vi "Test Connection.vi"() -> ()   [LabVIEW 2020]
uses:
  <vilib>/LabVIEW Open Source Project/MQTT Client/Client class/Client.lvclass
  <vilib>/LabVIEW Open Source Project/MQTT Connection/MQTT_Base/Base Class/MQTT_Base.lvclass
  <vilib>/LabVIEW Open Source Project/MQTT Control Packets/Control Packets/PUBLISH/PUBLISH.lvclass
  <vilib>/LabVIEW Open Source Project/MQTT Control Packets/Control Packets/ControlPacket/ControlPacket.lvclass
  <vilib>/LabVIEW Open Source Project/Connection/Connection.TCP/Connection.TCP.lvclass
  <vilib>/LabVIEW Open Source Project/Connection/Connection.LocalQueue/Connection.LocalQueue.lvclass
  <vilib>/LabVIEW Open Source Project/Connection/Connection/Connection.lvclass
  <vilib>/LabVIEW Open Source Project/MQTT Control Packets/Control Packets/CONNECT/ConnectFlags -- cluster.ctl
  <vilib>/LabVIEW Open Source Project/MQTT Control Packets/Control Packets/CONNECT/CONNECT.lvclass
  Class/SecureMqttCodec/SecureMqttCodec.lvclass
  <vilib>/LabVIEW Open Source Project/MQTT Control Packets/Control Packets/ControlPacket/QualityOfService -- enum.ctl
  C:/Program Files/National Instruments/LabVIEW 2020/vi.lib/LabVIEW Open Source Project/Connection/Connection/Connection.lvclass
  C:/Program Files/National Instruments/LabVIEW 2020/vi.lib/LabVIEW Open Source Project/Connection/Connection.TCP/Connection.TCP.lvclass
  C:/Program Files/National Instruments/LabVIEW 2020/vi.lib/LabVIEW Open Source Project/MQTT Connection/MQTT_Base/Base Class/MQTT_Base.lvclass
  C:/Program Files/National Instruments/LabVIEW 2020/vi.lib/LabVIEW Open Source Project/MQTT Client/Client class/Client.lvclass
  C:/Program Files/National Instruments/LabVIEW 2020/vi.lib/LabVIEW Open Source Project/Connection/Connection.LocalQueue/Connection.LocalQueue.lvclass
  C:/Program Files/National Instruments/LabVIEW 2020/vi.lib/LabVIEW Open Source Project/MQTT Control Packets/Control Packets/ControlPacket/ControlPacket.lvclass
  C:/Program Files/National Instruments/LabVIEW 2020/vi.lib/LabVIEW Open Source Project/MQTT Control Packets/Control Packets/PUBLISH/PUBLISH.lvclass
panel:
  out "Incoming Message":u8[](array[numeric]) format="%08b"
  in  "Subscribe":bool
  out "Suback":bool
  out "Published":bool
  in  "Publish":bool
  in  "Stop Client":bool
  out "error out":errorcluster
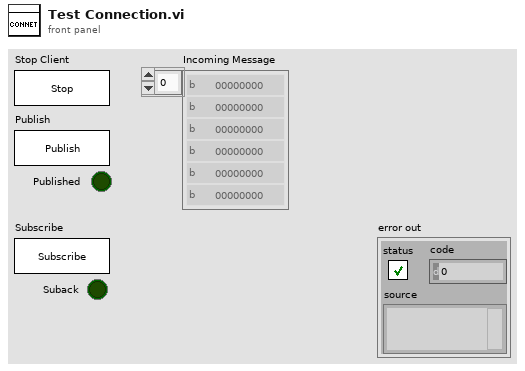
[diagram p1: front panel]
types:
  T1 = typedef "MQTT_Control_Packets.lvlib/CONNECT.lvclass/ConnectFlags -- cluster.ctl" = cluster{"Reserved":bool, "Clean Session":bool, "Will Flag":bool, "Will QoS 1":bool, "Will QoS 2":bool, "Will Retain":bool, "Password Flag":bool, "User Name Flag":bool}
  T2 = cluster{"Will Topic":string, "Will Message":string, "Username":string, "Password":string}
  T3 = typedef "MQTT Client.lvlib/Client.lvclass/Public Events -- cluster.ctl" = cluster{"Connection Status":refnum<user-event>, "Connected":refnum<user-event>, "Application Message":refnum<user-event>}
  T4 = typedef "MQTT Base.lvlib/MQTT_Base.lvclass/Public Events -- cluster.ctl" = cluster{"Stop Event":refnum<user-event>, "Error Event":refnum<user-event>, "Inbound Message":refnum<user-event>}
  T5 = typedef "MQTT_Control_Packets.lvlib/ControlPacket.lvclass/QualityOfService -- enum.ctl" = enum16{"0 (At Most Once)", "1 (At Least Once)", "2 (Exactly Once)"}
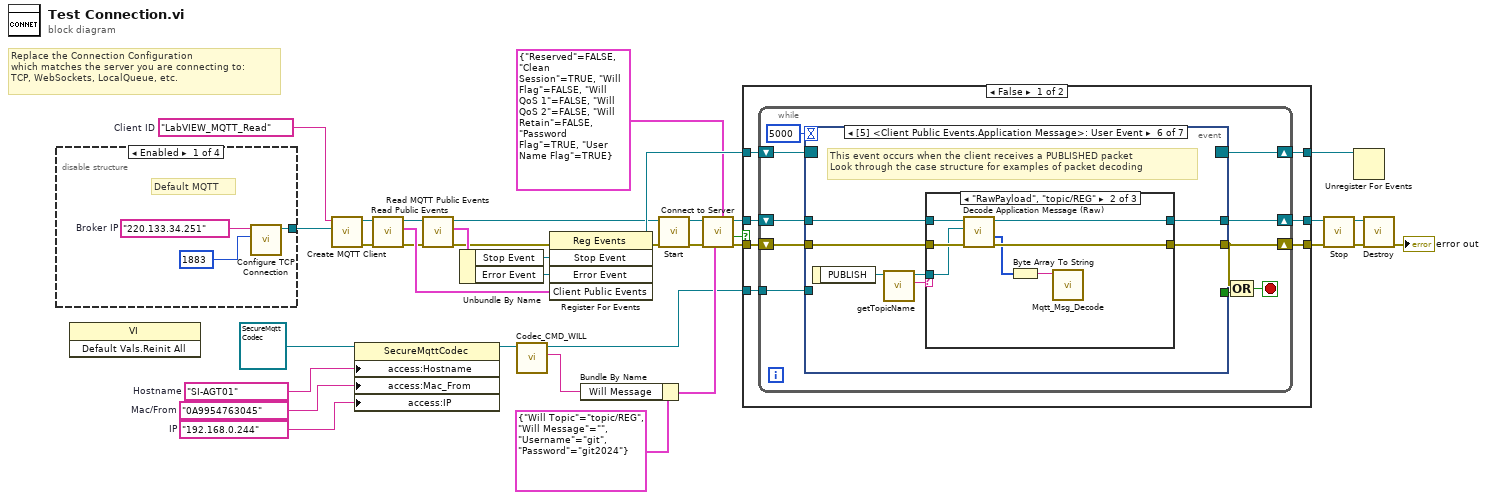
[diagram p0: block diagram]
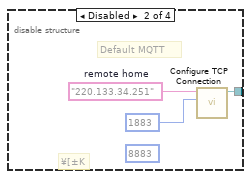
[diagram p2: hidden frame]
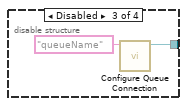
[diagram p3: hidden frame]
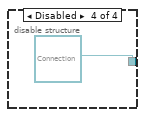
[diagram p4: hidden frame]
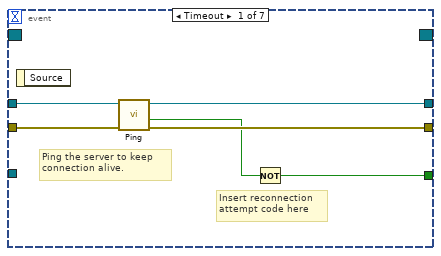
[diagram p5: hidden frame]
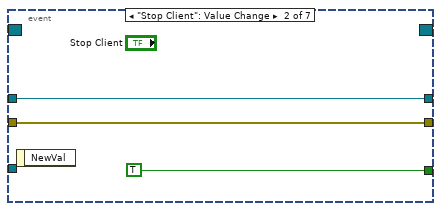
[diagram p6: hidden frame]
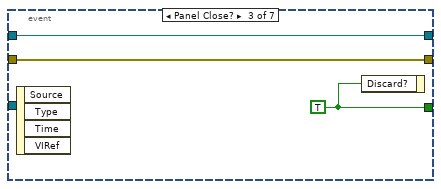
[diagram p7: hidden frame]
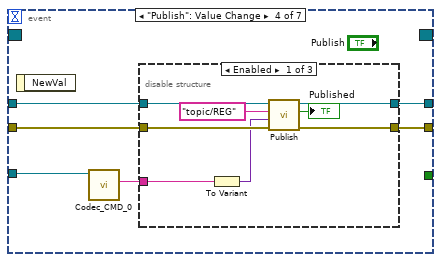
[diagram p8: hidden frame]
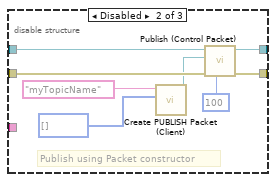
[diagram p9: hidden frame]
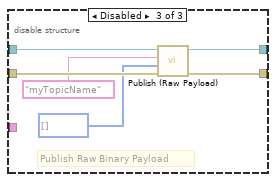
[diagram p10: hidden frame]
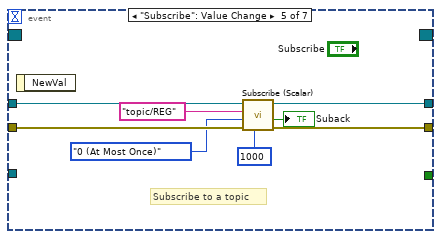
[diagram p11: hidden frame]
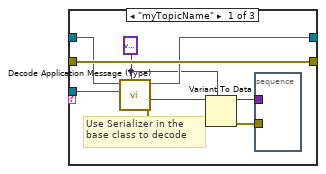
[diagram p12: hidden frame]
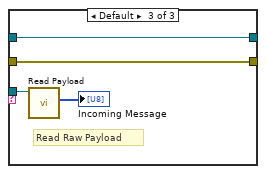
[diagram p13: hidden frame]
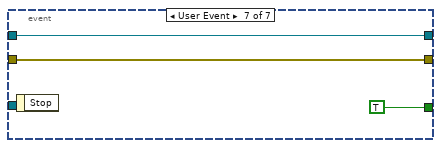
[diagram p14: hidden frame]
diagram:
  w1 = "192.168.0.244"  # IP
  w2 = "0A9954763045"  # Mac/From
  w3 = "SI-AGT01"  # Hostname
  w9 = "LabVIEW_MQTT_Read"  # Client ID
  # "Replace the Connection Configuration\nwhich matches the server you are connecting to:\nTCP, WebSockets, LocalQueue, etc."
  n1 = disable-structure shown="Enabled" {
    disable-tunnel: [w37 w40 w43 refnum<class "Connection.lvclass"> refnum ("Connection Configuration")] -> w35
    frame Enabled {
      w36 = "220.133.34.251"  # Broker IP
      # "Default MQTT"
      n2 = call <vilib>:"Configure TCP Connection.vi"("remote port (80)"=u16 1883, "address (localhost)"=w36) -> ("Connection.TCP"=w37:refnum<class "Connection.TCP.lvclass">)  [unwired: 8 in, 1 out]
    }
    frame Disabled {
      (unwired) u16 8883 ("remote port (80)")
      w39 = "220.133.34.251"  # remote home
      # "¥[±K"
      # "Default MQTT"
      n3 = call <vilib>:"Configure TCP Connection.vi"("remote port (80)"=u16 1883, "address (localhost)"=w39) -> ("Connection.TCP"=w40:refnum<class "Connection.TCP.lvclass">)  [unwired: 8 in, 1 out]
    }
    frame Disabled {
      n4 = call <vilib>:"Configure Queue Connection.vi"("Queue Name"="queueName") -> ("Connection.LocalQueue"=w43:refnum<class "Connection.LocalQueue.lvclass">)  [unwired: 9 in, 1 out]
    }
    frame Disabled {
    }
  }
  n5 = invoke class="VI" method="Default Vals.Reinit All"() -> ()  [unwired: 3 in, 3 out]
  n6 = call <vilib>:"Create MQTT Client.vi"("Connection Configuration"=w35, "ID (empty:generate new)"=w9) -> ("error out"=w14:errorcluster, "Client out"=w12:refnum<class "Client.lvclass">)  [unwired: 8 in]
  n7 = property class="SecureMqttCodec"(reference=refnum<class "SecureMqttCodec.lvclass"> refnum ("SecureMqttCodec.lvclass"), "access:Hostname"=w3, "access:Mac_From"=w2, "access:IP"=w1) -> (reference out=w4:refnum<class "SecureMqttCodec.lvclass">)  [unwired: 1 in, 1 out]
  n8 = call <vilib>:"Read Public Events.vi"("error in (no error)"=w14, "Client in"=w12) -> ("error out"=w15:errorcluster, "Client Public Events"=w17:T3, "Client out"=w13:refnum<class "Client.lvclass">)  [unwired: 7 in]
  n9 = call <vilib>:"Read MQTT Public Events.vi"("error in (no error)"=w15, "MQTT_Base in"=w13) -> ("error out"=w16:errorcluster, "MQTT Public Events"=w29:T4, "MQTT_Base out"=w19:refnum<class "Client.lvclass">)  [unwired: 7 in]
  n10 = Unbundle By Name(w29) -> ("Stop Event"=w27:refnum<user-event>, "Error Event"=w28:refnum<user-event>)
  n11 = call "Codec_CMD_WILL.vi"("SecureMqttCodec in"=w4) -> ("<JSON>"=w6:string, "SecureMqttCodec out"=w5:refnum<class "SecureMqttCodec.lvclass">)  [unwired: 8 in, 1 out]
  n12 = register-events(error in=w16, w27, w28, w17) -> (reference out=w22:refnum<event-registration>, error out=w18:errorcluster)  [unwired: 1 in]
  n13 = Bundle By Name(cluster=T2 {"Will Topic"="topic/REG", "Will Message"="", "Username"="git", "Password"="git2024"} ("Payload"), "Will Message"=w6) -> (w8:T2)
  n14 = call <vilib>:"Start.vi"("error in (no error)"=w18, "MQTT_Base in"=w19) -> ("error out"=w21:errorcluster, "MQTT_Base out"=w20:refnum<class "Client.lvclass">)  [unwired: 7 in, 1 out]
  n15 = call <vilib>:"Connect to Server.vi"("Connect Flags"=T1 {"Reserved"=FALSE, "Clean Session"=TRUE, "Will Flag"=FALSE, "Will QoS 1"=FALSE, "Will QoS 2"=FALSE, "Will Retain"=FALSE, "Password Flag"=TRUE, "User Name Flag"=TRUE}, "Payload"=w8, "error in (no error)"=w21, "Client in"=w20) -> ("error out"=w25:errorcluster, "timed out"=w24:bool, "Client out"=w26:refnum<class "Client.lvclass">)  [unwired: 4 in, 1 out]
  n16 = case shown="False" w24 {
    tunnel: w22 -> [w51 w142]
    tunnel: [w50 w142] -> w23
    tunnel: w25 -> [w47 w140]
    tunnel: w26 -> [w49 w141]
    tunnel: [w48 w141] -> w31
    tunnel: [w46 w140] -> w33
    tunnel: w5 -> [w45 _]
    frame False {
      n17 = while {
        shift-right: [w60] -> w50
        shift-left: w51 -> [w61]
        shift-right: [w53] -> w48
        shift-left: w49 -> [w54]
        shift-right: [w58] -> w46
        shift-left: w47 -> [w59]
        tunnel: w45 -> [w52]
        stop <- w57 stop-if-true
        n18 = event shown="[5] <Client Public Events.Application Message>: User Event" {
          selector: w61 -> [_ _ _ _ _ _ _]
          dyn-events: [_ _ _ _ _ _ _] -> w60
          timeout: 5000 -> [_ _ _ _ _ _ _]
          tunnel: w59 -> [w66 w69 w71 w78 w107 w112 w139]
          tunnel: [w64 w69 w71 w77 w106 w113 w139] -> w58
          tunnel: [w63 TRUE w73 _ _ _ TRUE] -> w56
          tunnel: w54 -> [w67 w70 w72 w79 w109 w115 w137]
          tunnel: [w65 w70 w72 w76 w105 w114 w137] -> w53
          tunnel: w52 -> [_ _ _ w75 _ _ _]
          event Timeout {
            # "Insert reconnection\nattempt code here"
            # "Ping the server to keep\nconnection alive."
            n19 = event-data() -> ()  [unwired: 1 in, 1 out]
            n20 = call <vilib>:"Ping.vi"("error in (no error)"=w66, "Client in"=w67) -> ("error out"=w64:errorcluster, "Server responded"=w62:bool, "Client out"=w65:refnum<class "Client.lvclass">)  [unwired: 6 in, 1 out]
            n21 = Not(x=w62) -> (.not. x?=w63:bool)
          }
          event "Stop Client": Value Change {
            n22 = event-data() -> ()  [unwired: 1 in, 1 out]
          }
          event Panel Close? {
            w73 = TRUE
            n23 = event-data() -> ()  [unwired: 1 in, 4 out]
            n24 = event-data("Discard?"=w73) -> ()  [unwired: 1 in, 1 out]
          }
          event "Publish": Value Change {
            n25 = event-data() -> ()  [unwired: 1 in, 1 out]
            n26 = call "Codec_CMD_0.vi"("SecureMqttCodec in"=w75) -> ("<JSON>"=w74:string)  [unwired: 8 in, 2 out]
            n27 = disable-structure shown="Enabled" {
              disable-tunnel: w79 -> [w87 w93 w101]
              disable-tunnel: w78 -> [w86 w91 w98]
              disable-tunnel: [w85 w90 w99] -> w77
              disable-tunnel: [w84 w92 w100] -> w76
              disable-tunnel: w74 -> [w80 _ _]
              frame Enabled {
                n28 = To Variant(anything=w80) -> (Variant=w82:variant)
                n29 = call <vilib>:"Publish.vi"("error in (no error)"=w86, "Payload"=w82, "Topic Name (empty: Payload name)"="topic/REG", "Client in"=w87) -> ("error out"=w85:errorcluster, "Published"=→"Published":bool, "Client out"=w84:refnum<class "Client.lvclass">)  [unwired: 5 in]
              }
              frame Disabled {
                # "Publish using Packet constructor"
                n30 = call <vilib>:"Create PUBLISH Packet (Client).vi"("Payload"=u8[] [], "Topic Name"="myTopicName" ("Topic Name (empty: Payload name)")) -> ("PUBLISH"=w88:refnum<class "PUBLISH.lvclass">)  [unwired: 6 in, 3 out]
                n31 = call <vilib>:"Publish (Control Packet).vi"("timeout (1000ms)"=100 ("timeout (0ms : no ack)"), "error in (no error)"=w91, "PUBLISH"=w88, "Client in"=w93) -> ("error out"=w90:errorcluster, "Client out"=w92:refnum<class "Client.lvclass">)  [unwired: 5 in, 1 out]
              }
              frame Disabled {
                # "Publish Raw Binary Payload"
                n32 = call <vilib>:"Publish (Raw Payload).vi"("error in (no error)"=w98, "Binary Payload"=u8[] [] ("Payload"), "Topic Name"="myTopicName" ("Topic Name (empty: Payload name)"), "Client in"=w101) -> ("error out"=w99:errorcluster, "Client out"=w100:refnum<class "Client.lvclass">)  [unwired: 5 in, 1 out]
              }
            }
          }
          event "Subscribe": Value Change {
            # "Subscribe to a topic"
            n33 = event-data() -> ()  [unwired: 1 in, 1 out]
            n34 = call <vilib>:"Subscribe (Scalar).vi"("timeout (1000ms)"=1000 ("timeout (100ms)"), "error in (no error)"=w107, "QoS"=QualityOfService_--_enum."0 (At Most Once)", "Topic Filter"="topic/REG" ("Topic Name (empty: Payload name)"), "Client in"=w109) -> ("error out"=w106:errorcluster, "Ack"=→"Suback":bool, "Client out"=w105:refnum<class "Client.lvclass">)  [unwired: 4 in]
          }
          event User Event {
            # "This event occurs when the client receives a PUBLISHED packet\nLook through the case structure for examples of packet decoding"
            n35 = event-data() -> ("PUBLISH"=w110:refnum<class "PUBLISH.lvclass">)  [unwired: 1 in]
            n36 = call <vilib>:"getTopicName.vi"("PUBLISH in"=w110) -> ("Topic"=w116:string, "PUBLISH out"=w111:refnum<class "PUBLISH.lvclass">)  [unwired: 8 in, 1 out]
            n37 = case shown="\"RawPayload\", \"topic/REG\"" w116 {
              tunnel: w115 -> [w122 w132 w136]
              tunnel: [w121 w131 w136] -> w114
              tunnel: [w125 w130 w135] -> w113
              tunnel: w112 -> [w125 w129 w135]
              tunnel: w111 -> [w120 w128 w134]
              frame "myTopicName" {
                w118 = variant ("Type")
                # "Use Serializer in the\nbase class to decode"
                n38 = call <vilib>:"Decode Application Message (Type).vi"("Type"=w118, "PUBLISH"=w120, "Client in"=w122) -> ("error out"=w117:errorcluster, "Payload"=w119:variant, "Client out"=w121:refnum<class "Client.lvclass">)  [unwired: 5 in, 1 out]
                n39 = Variant To Data(error in=w117, type=w118, Variant=w119) -> (data=w124:variant, error out=w123:errorcluster)
                n40 = stacked-sequence {
                  tunnel: w124 -> [_]
                  tunnel: w123 -> [_]
                  frame #0 {
                  }
                }
              }
              frame "RawPayload", "topic/REG" {
                n41 = call <vilib>:"Decode Application Message (Raw).vi"("error in (no error)"=w129, "PUBLISH"=w128, "Client in"=w132) -> ("error out"=w130:errorcluster, "Payload"=w127:u8[], "Client out"=w131:refnum<class "Client.lvclass">)  [unwired: 5 in, 1 out]
                n42 = Byte Array To String(unsigned byte array=w127) -> (string=w126:string)
                n43 = call "Mqtt_Msg_Decode.vi"("CMD_Response"=w126) -> ()  [unwired: 9 in, 2 out]
              }
              frame Default {
                # "Read Raw Payload"
                n44 = call <vilib>:"Read Payload.vi"("ControlPacket in"=w134) -> ("Payload"=→"Incoming Message":u8[])  [unwired: 9 in, 1 out]
              }
            }
          }
          event User Event {
            n45 = event-data() -> ()  [unwired: 1 in, 1 out]
          }
        }
        n46 = Compound Arithmetic op=OR(w58, w56) -> (w57:bool)
      }
    }
    frame True {
    }
  }
  n47 = call <vilib>:"Stop.vi"("error in (no error)"=w33, "MQTT_Base in"=w31) -> ("error out"=w32:errorcluster, "MQTT_Base out"=w30:refnum<class "Client.lvclass">)  [unwired: 7 in, 1 out]
  n48 = Unregister For Events(event registration refnum=w23) -> ()  [unwired: 1 in, 1 out]
  n49 = call <vilib>:"Destroy.vi"("error in (no error)"=w32, "MQTT_Base in"=w30) -> ("error out"=→"error out":errorcluster)  [unwired: 8 in, 1 out]
